vi "temp.vi"   [LabVIEW 2017]
uses:
  Configuration/Controls/Config Data.ctl
types:
  T1 = typedef "Config Data.ctl" = cluster{"Door Open":dbl, "Door Close":dbl, "Travel Time":dbl, "Inactivity Time":dbl}
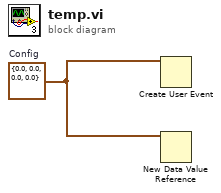
[diagram p0: block diagram]
diagram:
  w1 = T1 {"Door Open"=0.0, "Door Close"=0.0, "Travel Time"=0.0, "Inactivity Time"=0.0}  # Config
  n1 = Create User Event(user event datatype=w1) -> ()  [unwired: 1 in, 2 out]
  n2 = New Data Value Reference(data value=w1) -> ()  [unwired: 1 in, 2 out]
